vi "IndexControl.vi"(8 "Power":dbl, 9 "Chamber":bool, 10 "Back":bool, 11 "Forward":bool) -> (2 "Numeric":dbl)   [LabVIEW 2011]
uses:
  <vilib>/Rock Robotics/WPI/Relay/WPI_RelayValue.ctl
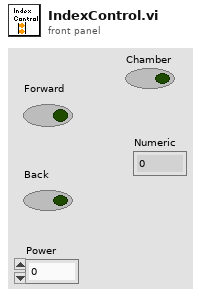
[diagram p1: front panel]
types:
  T1 = typedef "WPI_RelayDevRef.ctl" = cluster{"DevStatus":errorcluster, "Relay Channel":T2, "Digital Module":T3, "Relay Direction":T4}
  T2 = typedef "FPGA_DIORelayChannel.ctl" = enum8{"Relay 1", "Relay 2", "Relay 3", "Relay 4", "Relay 5", "Relay 6", "Relay 7", "Relay 8", "Invalid"}
  T3 = typedef "FPGA_TypedefDigitalModule.ctl" = enum16{"Digital Module 1", "Digital Module 2"}
  T4 = typedef "WPI_RelayDirection.ctl" = enum16{"Both directions", "Forward only", "Reverse only"}
  T5 = typedef "WPI_RelayValue.ctl" = enum16{"Off", "On", "Forward", "Reverse"}
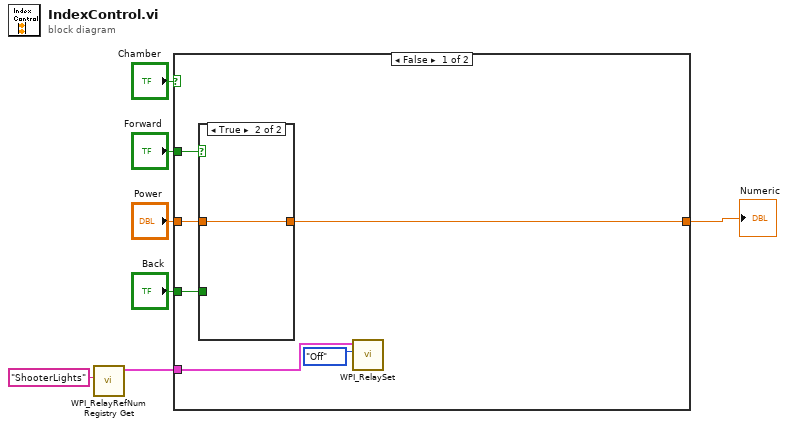
[diagram p0: block diagram]
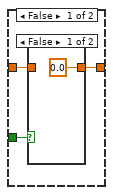
[diagram p2: hidden frame]
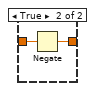
[diagram p3: hidden frame]
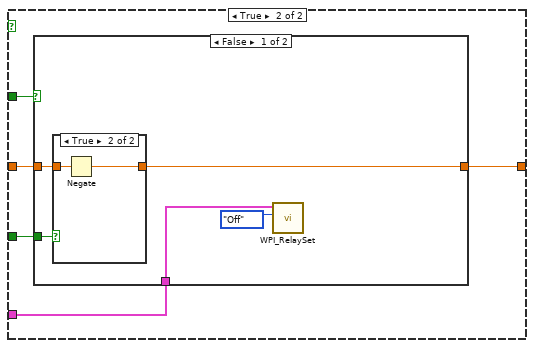
[diagram p4: hidden frame]
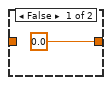
[diagram p5: hidden frame]
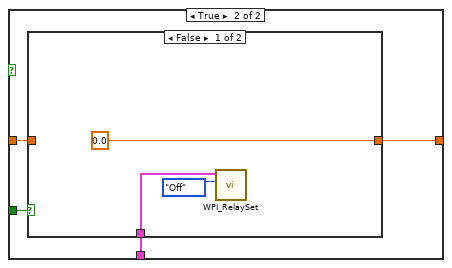
[diagram p6: hidden frame]
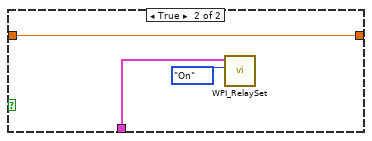
[diagram p7: hidden frame]
diagram:
  n1 = call <vilib>:"WPI_RelayRefNum Registry Get.vi"("refnum name"="ShooterLights") -> ("RelayDevRef"=w1:T1)  [unwired: 9 in, 1 out]
  n2 = case shown="False" "Chamber" {
    tunnel: "Forward" -> [w13 w23]
    tunnel: "Power" -> [w12 w24]
    tunnel: [w11 w25] -> w5
    tunnel: "Back" -> [w10 w22]
    tunnel: w1 -> [w9 w21]
    frame False {
      n3 = case shown="True" w13 {
        tunnel: w12 -> [w15 w20]
        tunnel: [w14 w20] -> w11
        tunnel: w10 -> [w16 _]
        frame False {
          n4 = case shown="False" w16 {
            tunnel: w15 -> [_ w18]
            tunnel: [0.0 w19] -> w14
            frame False {
            }
            frame True {
              n5 = Negate(x=w18) -> (-x=w19:dbl)
            }
          }
        }
        frame True {
        }
      }
      n6 = call <vilib>:"WPI_RelaySet.vi"("RelayValue"=WPI_RelayValue."Off", "RelayDevRef"=w9) -> ()  [unwired: 8 in, 2 out]
    }
    frame True {
      n7 = case shown="False" w23 {
        tunnel: w24 -> [w30 w36]
        tunnel: [w29 w37] -> w25
        tunnel: w22 -> [w28 w35]
        tunnel: w21 -> [w27 w34]
        frame False {
          n8 = case shown="True" w28 {
            tunnel: w30 -> [_ w32]
            tunnel: [0.0 w33] -> w29
            frame False {
            }
            frame True {
              n9 = Negate(x=w32) -> (-x=w33:dbl)
            }
          }
          n10 = call <vilib>:"WPI_RelaySet.vi"("RelayValue"=WPI_RelayValue."Off", "RelayDevRef"=w27) -> ()  [unwired: 8 in, 2 out]
        }
        frame True {
          n11 = case shown="False" w35 {
            tunnel: [0.0 w43] -> w37
            tunnel: w36 -> [_ w43]
            tunnel: w34 -> [w39 w42]
            frame False {
              n12 = call <vilib>:"WPI_RelaySet.vi"("RelayValue"=WPI_RelayValue."Off", "RelayDevRef"=w39) -> ()  [unwired: 8 in, 2 out]
            }
            frame True {
              n13 = call <vilib>:"WPI_RelaySet.vi"("RelayValue"=WPI_RelayValue."On", "RelayDevRef"=w42) -> ()  [unwired: 8 in, 2 out]
            }
          }
        }
      }
    }
  }
  "Numeric" <- w5
